vi "Send SwitchOption.vi"(4 "Message Priority":T1=enum."Normal", 6 "SubPanelRef":refnum<vi>, 7 "Message Enqueuer":refnum<class "Message Enqueuer.lvclass">, 8 "error in (no error)":errorcluster, 9 "Base Path":path, 10 "ThreadName(\"\")":string, 11 "Message Type":refnum<class "SwitchOption Msg.lvclass">) -> (0 "error out":errorcluster)   [LabVIEW 2015, in "User_Actor.lvlib" / "SwitchOption Msg.lvclass"]
doc: "This VI sends the message to an actor."
uses:
  SwitchOption Msg.lvclass
  <vilib>/ActorFramework/Message Enqueuer/Message Enqueuer.lvclass
  <vilib>/ActorFramework/Message Enqueuer/Message Priority.ctl
  SwitchOption Msg.lvclass/SwitchOption Msg.ctl
  <vilib>/ActorFramework/Message Enqueuer/Message Enqueuer.lvclass/Message Enqueuer.ctl
  <vilib>/ActorFramework/Message Priority Queue/Priority Enqueue.vi
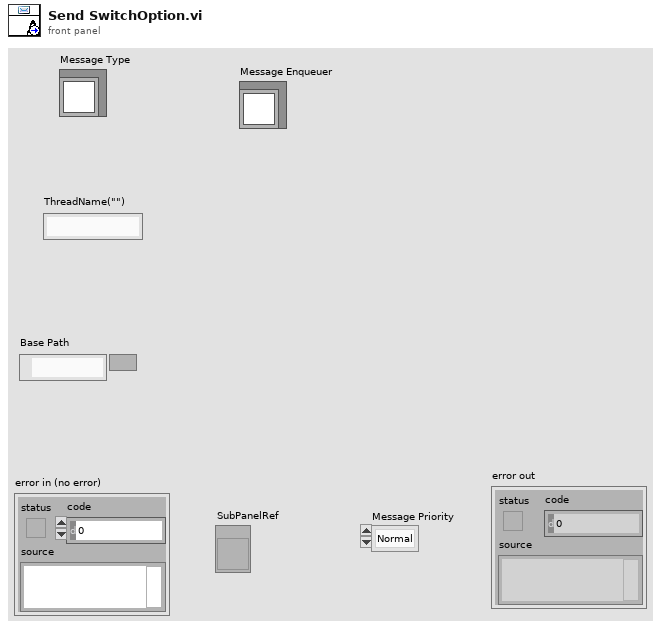
[diagram p1: front panel]
types:
  T1 = typedef "Actor Framework.lvlib/Message Enqueuer.lvclass/Message Priority.ctl" = enum16{"Low", "Normal", "High"}
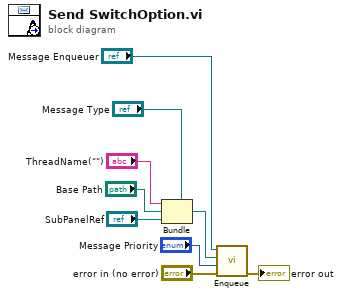
[diagram p0: block diagram]
diagram:
  n1 = Bundle(cluster="Message Type", "ThreadName(\"\")", "Base Path", "SubPanelRef") -> (w5:refnum<class "SwitchOption Msg.lvclass">)
  n2 = call <vilib>:"Enqueue.vi"("error in (no error)"="error in (no error)", "Message Priority (Normal)"="Message Priority", "Message"=w5, "Message Enqueuer in"="Message Enqueuer") -> ("error out"=→"error out":errorcluster)  [unwired: 6 in, 1 out]
